vi "Write Pulse Configuration.vi"(8 "error in (no error)":errorcluster, 10 "Configuration":T1={"Post-trigger delay"=0.01, "Post-trigger duration"=0.1, "Rate"=1000000.0, "Ranges"=[10.0], "Re-name channels"=[], "Active channels"="0:1", "External clock"=FALSE} {"Rate" format="%#_8pHz"; "Post-trigger duration" format="%#_6ps"; "Post-trigger delay" format="%#_6ps"; "Ranges" format="%#_6pV"}, 11 "NI-Scope Lock-in Driver in":refnum<class "NI-Scope Lock-in Driver.lvclass">) -> (0 "error out":errorcluster, 3 "NI-Scope Lock-in Driver out":refnum<class "NI-Scope Lock-in Driver.lvclass">)   [LabVIEW 2021, in "NI-Scope Lock-in Driver.lvclass"]
uses:
  NI-Scope Lock-in Driver.lvclass
  Instruments/Pulse Driver/Pusle Driver Configuration.ctl
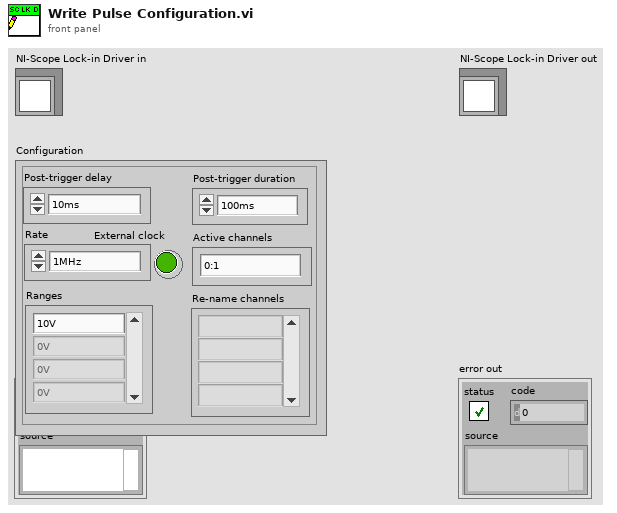
[diagram p1: front panel]
types:
  T1 = typedef "Pusle Driver Configuration.ctl" = cluster{"Post-trigger delay":dbl, "Post-trigger duration":dbl, "Rate":dbl, "Ranges":dbl[], "Re-name channels":string[], "Active channels":string, "External clock":bool}
  T2 = typedef "NI-Scope Lock-in Configuration.ctl" = cluster{"Points per sine wave":i32, "Rate":dbl, "Re-name channels":string[], "Active channels":string, "Ranges":dbl[], "Sync on trigger":bool, "R-Q":bool}
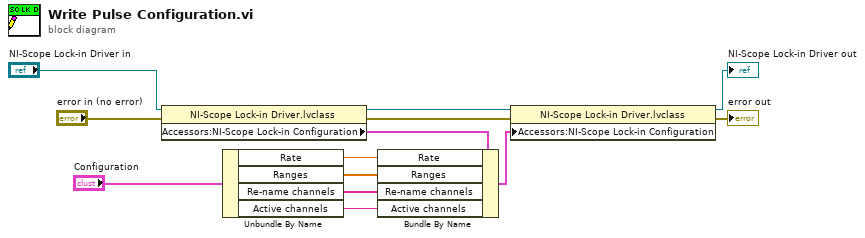
[diagram p0: block diagram]
diagram:
  n1 = property class="NI-Scope Lock-in Driver.lvclass"(reference="NI-Scope Lock-in Driver in", error in="error in (no error)") -> (reference out=w9:refnum<class "NI-Scope Lock-in Driver.lvclass">, error out=w12:errorcluster, "Accessors:NI-Scope Lock-in Configuration"=w7:T2)
  n2 = Unbundle By Name("Configuration") -> ("Rate"=w4:dbl, "Ranges"=w3:dbl[], "Re-name channels"=w2:string[], "Active channels"=w1:string)
  n3 = Bundle By Name(cluster=w7, "Rate"=w4, "Ranges"=w3, "Re-name channels"=w2, "Active channels"=w1) -> (w6:T2)
  n4 = property class="NI-Scope Lock-in Driver.lvclass"(reference=w9, error in=w12, "Accessors:NI-Scope Lock-in Configuration"=w6) -> (reference out=→"NI-Scope Lock-in Driver out":refnum<class "NI-Scope Lock-in Driver.lvclass">, error out=→"error out":errorcluster)
